vi "Shutdown.vi"(0 "reference in":refnum<class "DUT_Handler_Base.lvclass">, 5 "error in (no error)":errorcluster) -> (14 "reference in":refnum<class "DUT_Handler_Base.lvclass">, 19 "error out":errorcluster)   [LabVIEW 2022 SP3, in "DUT_Handler_Base.lvlib" / "DUT_Handler_Base.lvclass"]
uses:
  DUT_Handler_Base.lvclass
  EventData.ctl
  Action.ctl
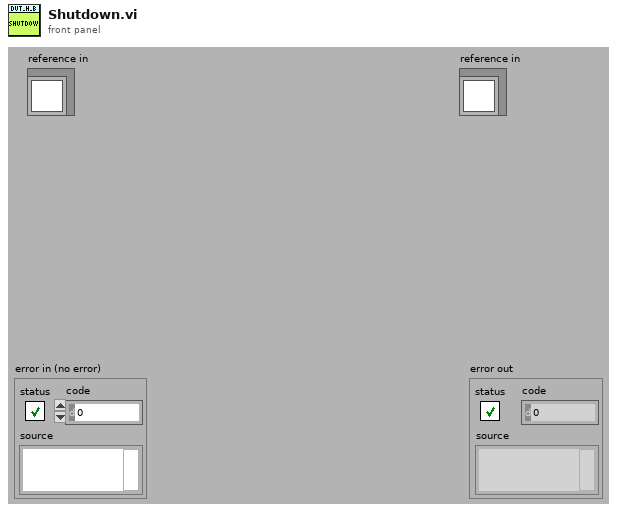
[diagram p1: front panel]
types:
  T1 = typedef "DUT_Handler_Base.lvlib/DUT_Handler_Base.lvclass/EventData.ctl" = cluster{"Action":T2, "SN":string, "BN":string, "DUT__ID":u32, "Message":string, "From":string, "To":string}
  T2 = typedef "DUT_Handler_Base.lvlib/DUT_Handler_Base.lvclass/Action.ctl" = enum16{"Load", "Cancel", "MoveIn", "MoveOut", "Abort", "Msg", "Enabled", "Disabled", "Fault", "Shutdown"}
  T3 = typedef "DUT_Handler_Base.lvlib/DUT_Handler_Base.lvclass/ObjectAttributes.ctl" = cluster{"Config":T4, "Event":refnum<user-event>}
  T4 = typedef "DUT_Handler_Base.lvlib/DUT_Handler_Base.lvclass/Config.ctl" = cluster{"default":string}
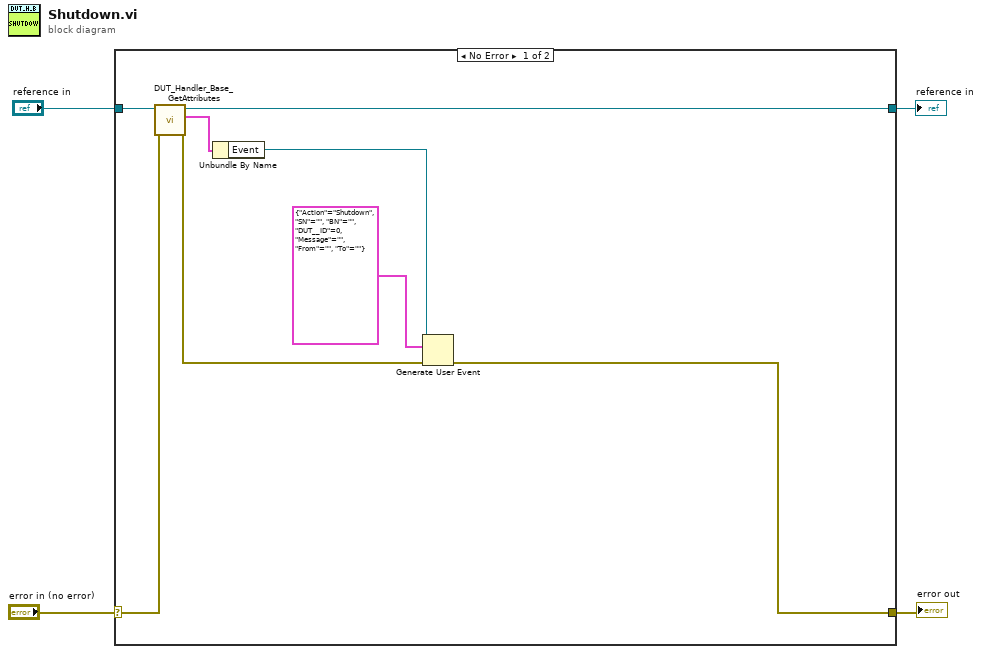
[diagram p0: block diagram]
diagram:
  n1 = case shown="No Error" "error in (no error)" {
    selector: "error in (no error)" -> [w12 w14]
    tunnel: [w6 w14] -> w3
    tunnel: [w9 w13] -> w1
    tunnel: "reference in" -> [w10 w13]
    frame No Error {
      n2 = call "DUT_Handler_Base_GetAttributes.vi"("error in (no error)"=w12, "reference in"=w10) -> ("error out"=w7:errorcluster, "Data"=w11:T3, "reference out"=w9:refnum<class "DUT_Handler_Base.lvclass">)  [unwired: 6 in, 1 out]
      n3 = Unbundle By Name(w11) -> ("Event"=w8:refnum<user-event>)
      n4 = Generate User Event(user event=w8, event data cluster=T1 {"Action"=enum."Shutdown", "SN"="", "BN"="", "DUT__ID"=0, "Message"="", "From"="", "To"=""} ("event data"), error in=w7) -> (error out=w6:errorcluster)  [unwired: 1 in, 1 out]
    }
    frame Error {
    }
  }
  "error out" <- w3
  "reference in" <- w1
